vi "Nested Unique.vi"(10 "Nested Alias":string, 11 "jettl Queue Actor in":refnum<class "jettl Queue Actor.lvclass">) -> (2 "Nested Alias Unique?":bool)   [LabVIEW 2021, in "jettl.lvlib" / "jettl Queue Actor.lvlib" / "jettl Queue Actor.lvclass"]
uses:
  jettl Queue Actor.lvclass
  jettl Queue Actor.lvclass/jettl Queue Actor.ctl
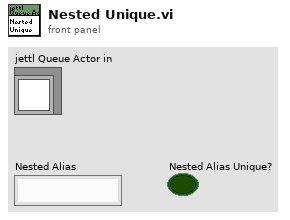
[diagram p1: front panel]
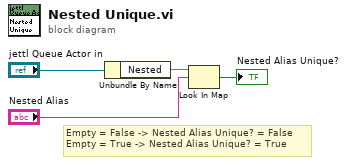
[diagram p0: block diagram]
diagram:
  # "Empty = False -> Nested Alias Unique? = False\nEmpty = True -> Nested Alias Unique? = True"
  n1 = Unbundle By Name("jettl Queue Actor in") -> ("Nested"=w2:map{string, refnum<data-value>})
  n2 = Look In Map(map=w2, key="Nested Alias") -> (key not found?=→"Nested Alias Unique?":bool)  [unwired: 1 in, 1 out]
